vi "Script on Test VI.vi"() -> ()   [LabVIEW 2016, in "SLL Scripting.lvlib"]
uses:
  SLL Scripting.lvlib
  <vilib>/Utility/traverseref.llb/TRef TravTarget.ctl
  <vilib>/Utility/traverseref.llb/VI Scripting - Traverse.lvlib
panel:
  out "Array 8":bool[](array[boolean])
  out "Array 7":string[](array[string])
  out "Array 6":string[][](array[string])
  out "Connected?":bool[](array[boolean])
  out "Source?":bool[](array[boolean])
  out "Array 5":string[](array[string])
  out "Array 4":string[](array[string])
  out "Array 3":string[](array[string])
  out "FP Class Names":string[](array[string])
  out "Array 2":string[](array[string])
  out "Array":bool[](array[boolean])
  out "BD Class Names":string[](array[string])
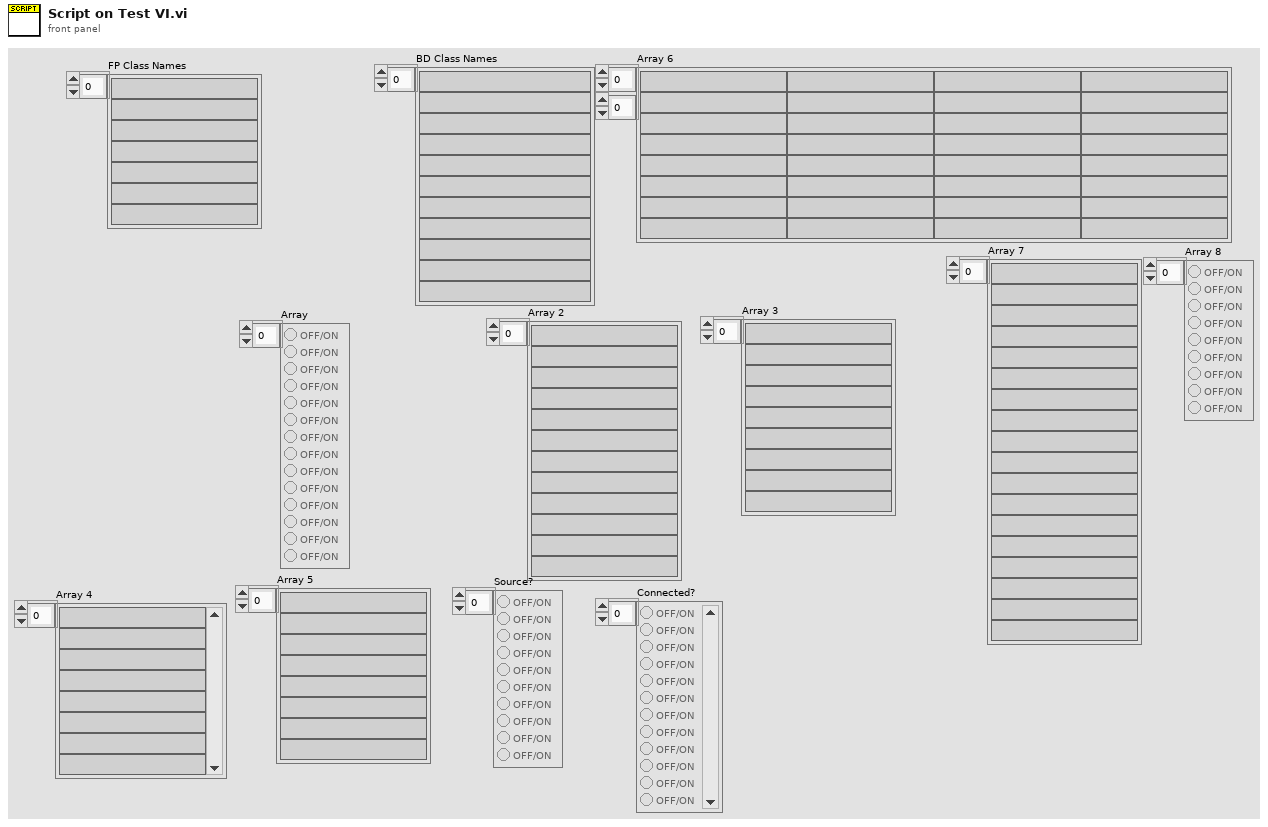
[diagram p1: front panel]
types:
  T1 = typedef "TRef TravTarget.ctl" = enum16{"FP", "BD", "Other"}
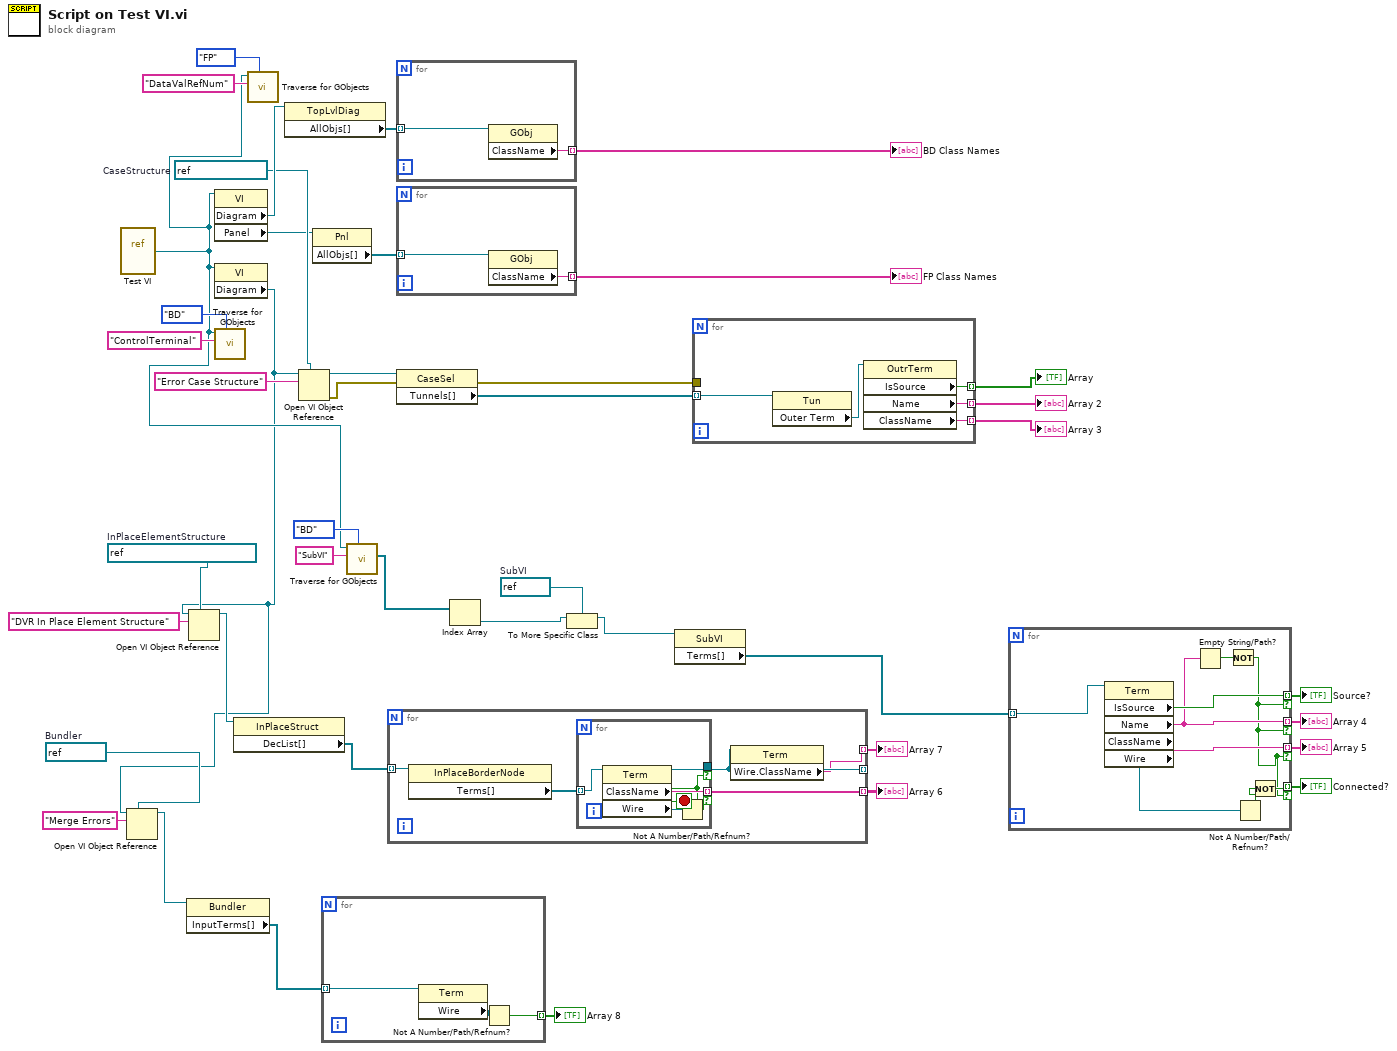
[diagram p0: block diagram]
diagram:
  w5 = refnum<vi> refnum  # Bundler
  w12 = refnum<vi> refnum  # InPlaceElementStructure
  w22 = refnum<vi> refnum  # SubVI
  w37 = refnum<vi> refnum  # CaseStructure
  n1 = vi-ref "Test VI.vi"() -> (w15:refnum<vi>)
  n2 = property class="VI"(reference=w15) -> ("Diagram"=w43:refnum<vi>, "Panel"=w32:refnum<vi>)  [unwired: 1 in, 2 out]
  n3 = property class="VI"(reference=w15) -> ("Diagram"=w4:refnum<vi>)  [unwired: 1 in, 2 out]
  n4 = Open VI Object Reference(7:w5, 10:"Merge Errors" ("name/order"), 11:w4) -> (3:w3:refnum<vi>)  [unwired: 1 in, 1 out]
  n5 = property class="Bundler"(reference=w3) -> ("InputTerms[]"=w2:refnum<vi>[])  [unwired: 1 in, 2 out]
  n6 = Open VI Object Reference(7:w12, 10:"DVR In Place Element Structure" ("name/order"), 11:w4) -> (3:w10:refnum<vi>)  [unwired: 1 in, 1 out]
  n7 = call <vilib>:"Traverse for GObjects.vi"("Traverse Target"=TRef_TravTarget."BD", "Class Name"="ControlTerminal", "VI Refnum"=w15) -> ()  [unwired: 5 in, 4 out]
  n8 = property class="InPlaceStruct"(reference=w10) -> ("DecList[]"=w9:refnum<vi>[])  [unwired: 1 in, 2 out]
  n9 = call <vilib>:"Traverse for GObjects.vi"("Traverse Target"=TRef_TravTarget."FP", "Class Name"="DataValRefNum", "VI Refnum"=w15) -> ()  [unwired: 5 in, 4 out]
  n10 = property class="TopLvlDiag"(reference=w43) -> ("AllObjs[]"=w42:refnum<vi>[])  [unwired: 1 in, 2 out]
  n11 = Open VI Object Reference(7:w37, 10:"Error Case Structure" ("name/order"), 11:w4) -> (0:w14:errorcluster, 3:w36:refnum<vi>)  [unwired: 1 in]
  n12 = property class="Pnl"(reference=w32) -> ("AllObjs[]"=w31:refnum<vi>[])  [unwired: 1 in, 2 out]
  n13 = for {
    tunnel: w2 -> [w46] mode=indexing
    tunnel: [w44] -> w1 mode=indexing
    n14 = property class="Term"(reference=w46) -> ("Wire"=w45:refnum<vi>)  [unwired: 1 in, 2 out]
    n15 = Not A Number/Path/Refnum?(number/path/refnum=w45) -> (NaN/Path/Refnum?=w44:bool)
  }
  "Array 8" <- w1
  n16 = call <vilib>:"Traverse for GObjects.vi"("Traverse Target"=TRef_TravTarget."BD", "Class Name"="SubVI", "VI Refnum"=w15) -> ("References"=w24:refnum<vi>[])  [unwired: 5 in, 3 out]
  n17 = for {
    tunnel: w9 -> [w51] mode=indexing
    tunnel: [w49] -> w8 mode=indexing
    tunnel: [w48] -> _ mode=indexing
    tunnel: [w47] -> w7 mode=indexing
    n18 = property class="InPlaceBorderNode"(reference=w51) -> ("Terms[]"=w50:refnum<vi>[])  [unwired: 1 in, 2 out]
    n19 = for {
      tunnel: w50 -> [w56] mode=indexing
      tunnel: [w55] -> w49 mode=indexing if=w52
      tunnel: [w53] -> w48 if=w52
      stop <- w52 stop-if-true
      n20 = property class="Term"(reference=w56) -> (reference out=w53:refnum<vi>, "ClassName"=w55:string, "Wire"=w54:refnum<vi>)  [unwired: 1 in, 1 out]
      n21 = Not A Number/Path/Refnum?(number/path/refnum=w54) -> (NaN/Path/Refnum?=w52:bool)
    }
    n22 = property class="Term"(reference=w48) -> ("Wire.ClassName"=w47:string)  [unwired: 1 in, 2 out]
  }
  "Array 6" <- w8
  "Array 7" <- w7
  n23 = for {
    tunnel: w42 -> [w58] mode=indexing
    tunnel: [w57] -> w41 mode=indexing
    n24 = property class="GObj"(reference=w58) -> ("ClassName"=w57:string)  [unwired: 1 in, 2 out]
  }
  "BD Class Names" <- w41
  n25 = for {
    tunnel: w31 -> [w60] mode=indexing
    tunnel: [w59] -> w30 mode=indexing
    n26 = property class="GObj"(reference=w60) -> ("ClassName"=w59:string)  [unwired: 1 in, 2 out]
  }
  "FP Class Names" <- w30
  n27 = property class="CaseSel"(reference=w36, error in=w14) -> (error out=w13:errorcluster, "Tunnels[]"=w35:refnum<vi>[])  [unwired: 1 out]
  n28 = Index Array(array=w24) -> (element=w23:refnum<vi>)  [unwired: 1 in]
  n29 = To More Specific Class(target class=w22, reference=w23) -> (specific class reference=w21:refnum<vi>)  [unwired: 1 in, 1 out]
  n30 = property class="SubVI"(reference=w21) -> ("Terms[]"=w20:refnum<vi>[])  [unwired: 1 in, 2 out]
  n31 = for {
    tunnel: w35 -> [w65] mode=indexing
    tunnel: [w63] -> w34 mode=indexing
    tunnel: [w62] -> w33 mode=indexing
    tunnel: [w61] -> w29 mode=indexing
    tunnel: w13 -> [_]
    n32 = property class="Tun"(reference=w65) -> ("Outer Term"=w64:refnum<vi>)  [unwired: 1 in, 2 out]
    n33 = property class="OutrTerm"(reference=w64) -> ("IsSource"=w63:bool, "Name"=w62:string, "ClassName"=w61:string)  [unwired: 1 in, 2 out]
  }
  "Array" <- w34
  "Array 2" <- w33
  "Array 3" <- w29
  n34 = for {
    tunnel: w20 -> [w72] mode=indexing
    tunnel: [w74] -> w17 mode=indexing if=w66
    tunnel: [w68] -> w19 mode=indexing if=w66
    tunnel: [w73] -> w18 mode=indexing if=w66
    tunnel: [w69] -> w16 mode=indexing if=w66
    n35 = property class="Term"(reference=w72) -> ("IsSource"=w74:bool, "Name"=w68:string, "ClassName"=w73:string, "Wire"=w71:refnum<vi>)  [unwired: 1 in, 2 out]
    n36 = Empty String/Path?(string/path=w68) -> (empty?=w67:bool)
    n37 = Not(x=w67) -> (.not. x?=w66:bool)
    n38 = Not A Number/Path/Refnum?(number/path/refnum=w71) -> (NaN/Path/Refnum?=w70:bool)
    n39 = Not(x=w70) -> (.not. x?=w69:bool)
  }
  "Array 4" <- w19
  "Array 5" <- w18
  "Source?" <- w17
  "Connected?" <- w16
